vi "Refresh Style data.vi"(8 "error in (no error)":errorcluster, 11 "Splitter in":refnum<class "Splitter.lvclass">) -> (0 "error out":errorcluster, 3 "Splitter out":refnum<class "Splitter.lvclass">)   [LabVIEW 2020, in "Splitter.lvclass"]
uses:
  Splitter.lvclass
  Splitter.lvclass/Splitter.ctl
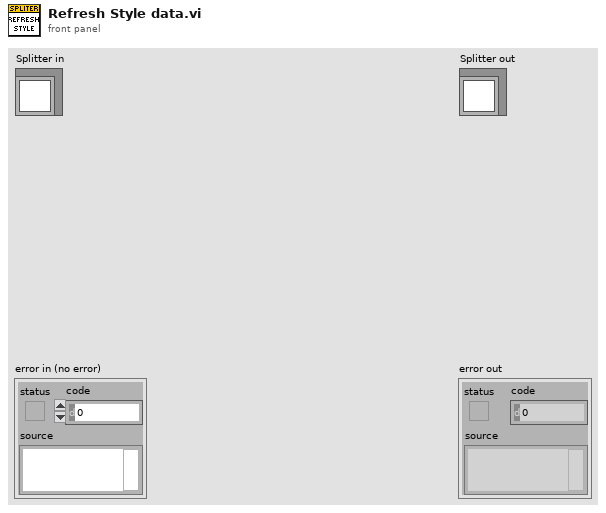
[diagram p1: front panel]
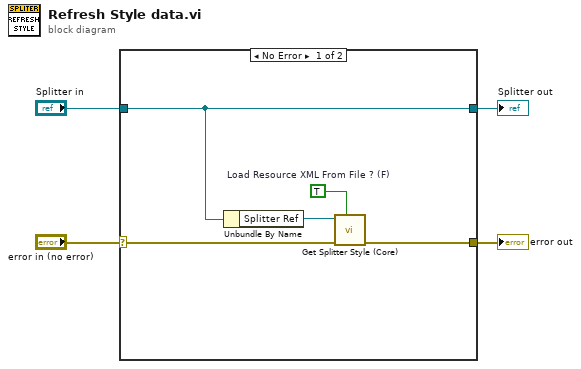
[diagram p0: block diagram]
diagram:
  n1 = case shown="No Error" "error in (no error)" {
    selector: "error in (no error)" -> [w8 w11]
    tunnel: [w7 w11] -> w3
    tunnel: [w9 w10] -> w1
    tunnel: "Splitter in" -> [w9 w10]
    frame No Error {
      w5 = TRUE  # Load Resource XML From File ? (F)
      n2 = Unbundle By Name(w9) -> ("Splitter Ref"=w6:refnum<vi>)
      n3 = call "Get Splitter Style (Core).vi"("Load Resource XML From File ? (F)"=w5, "error in (no error)"=w8, "Splitter in"=w6) -> ("error out"=w7:errorcluster)  [unwired: 5 in, 1 out]
    }
    frame Error {
    }
  }
  "error out" <- w3
  "Splitter out" <- w1
